vi "ACT_LabVIEW1_Task2B_Team072.vi"() -> ()   [LabVIEW 2016]
uses:
  <vilib>/express/express arith-compare/Formula/XNode/ExpressFormulaBlockNode.xnode
panel:
  out "RE":dbl
  in  "p (lb/in^3)":dbl
  in  "u (lb/(in*s))":dbl
  in  "L (in)":dbl
  in  "V (mi/hr)":dbl
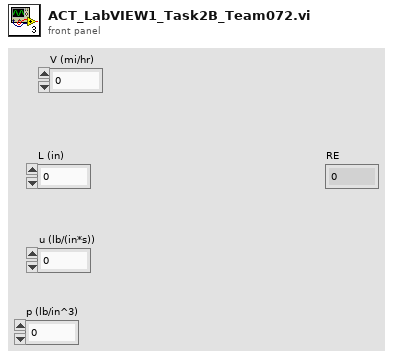
[diagram p1: front panel]
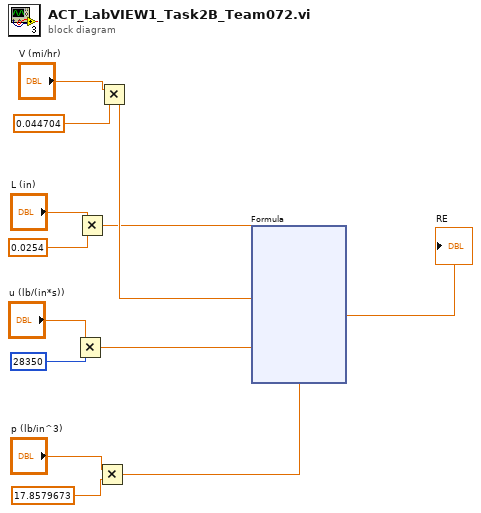
[diagram p0: block diagram]
diagram:
  n1 = Multiply(x="u (lb/(in*s))", y=28350) -> (x*y=w3:dbl)
  n2 = Multiply(x="L (in)", y=0.0254) -> (x*y=w4:dbl)
  n3 = Multiply(x="p (lb/in^3)", y=17.8579673) -> (x*y=w2:dbl)
  n4 = Multiply(x="V (mi/hr)", y=0.044704) -> (x*y=w5:dbl)
  n5 = xnode "Formula"("V"=w5, "L"=w4, "u"=w3, "p"=w2) -> ("Result"=→"RE":dbl)  [unwired: 1 in, 1 out]
